vi "High Resolution Timer Helper.vi"(8 "error in (no error)":errorcluster, 11 "Previous Time":dbl format="%_19f") -> (0 "error out":errorcluster, 2 "Time Difference (ms)":dbl format="%_19f", 3 "Current Time":dbl format="%_19f")   [LabVIEW 2018]
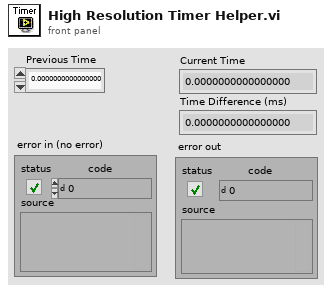
[diagram p1: front panel]
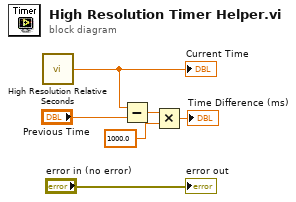
[diagram p0: block diagram]
diagram:
  n1 = call <vilib>:"High Resolution Relative Seconds.vi"() -> ("relative seconds"=w5:dbl)
  "Current Time" <- w5
  n2 = Subtract(x=w5, y="Previous Time") -> (x-y=w3:dbl)
  n3 = Multiply(x=w3, y=1000.0) -> (x*y=→"Time Difference (ms)":dbl)
  "error out" <- "error in (no error)"
